vi "Average_IBP_curves_baseline_fromFile.vi"() -> ()   [LabVIEW 2015]
panel:
  in  "file path dn":path
  out "Resampled i(B) array":dbl[][](array[numeric])
  out "Mean I(B)":dbl[](array[numeric])
  out "XY Graph":cluster{dbl[], "Array out":dbl[]}[](graph)
  in  "Counter":i8
  in  "Min Field (T)":dbl
  in  "dB (T)":dbl=0.0025
  in  "Max Field (T)":dbl=0.15
  out "B array":dbl[](array[numeric])
  in  "file path (dialog if empty)":path
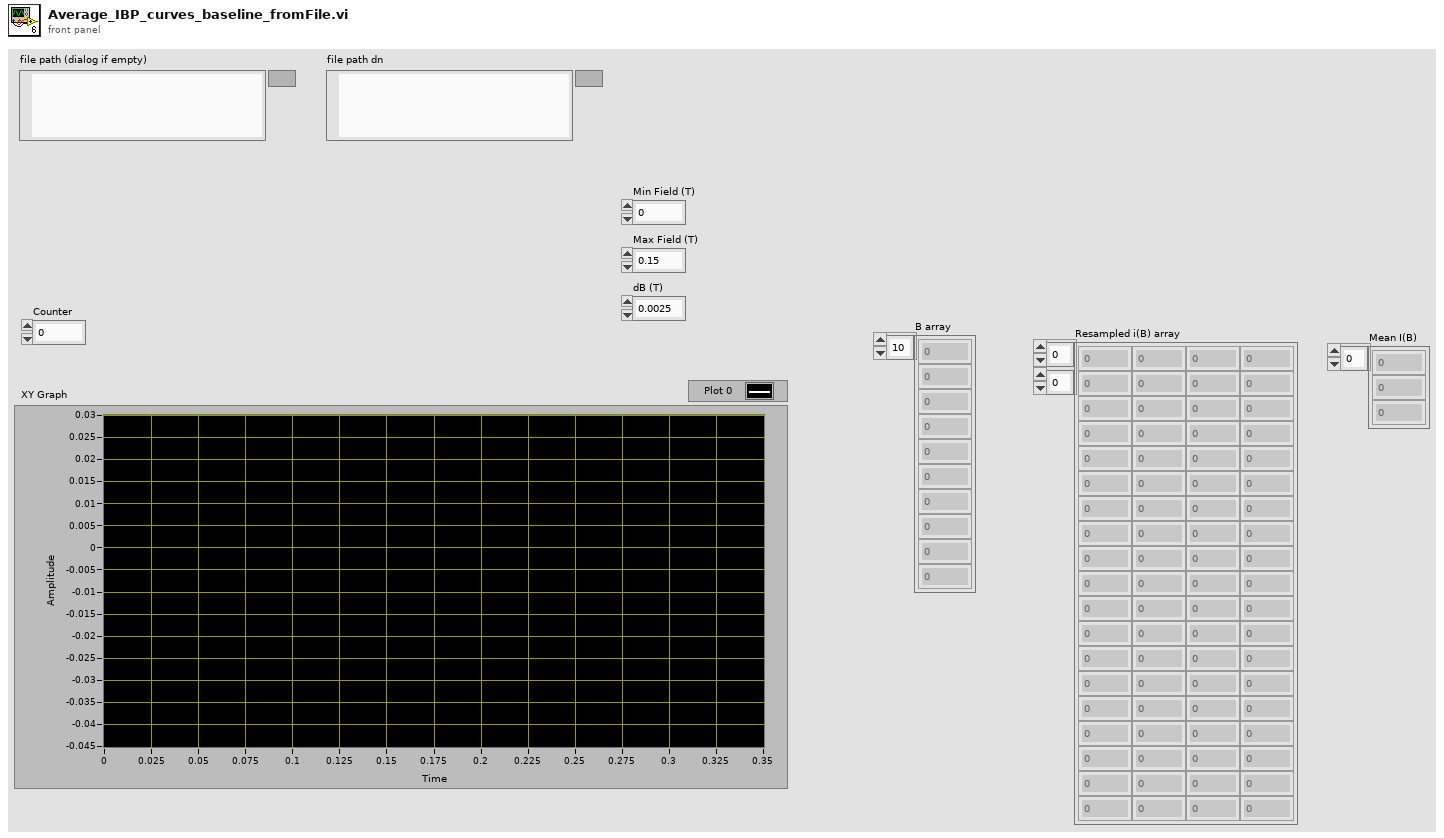
[diagram p1: front panel]
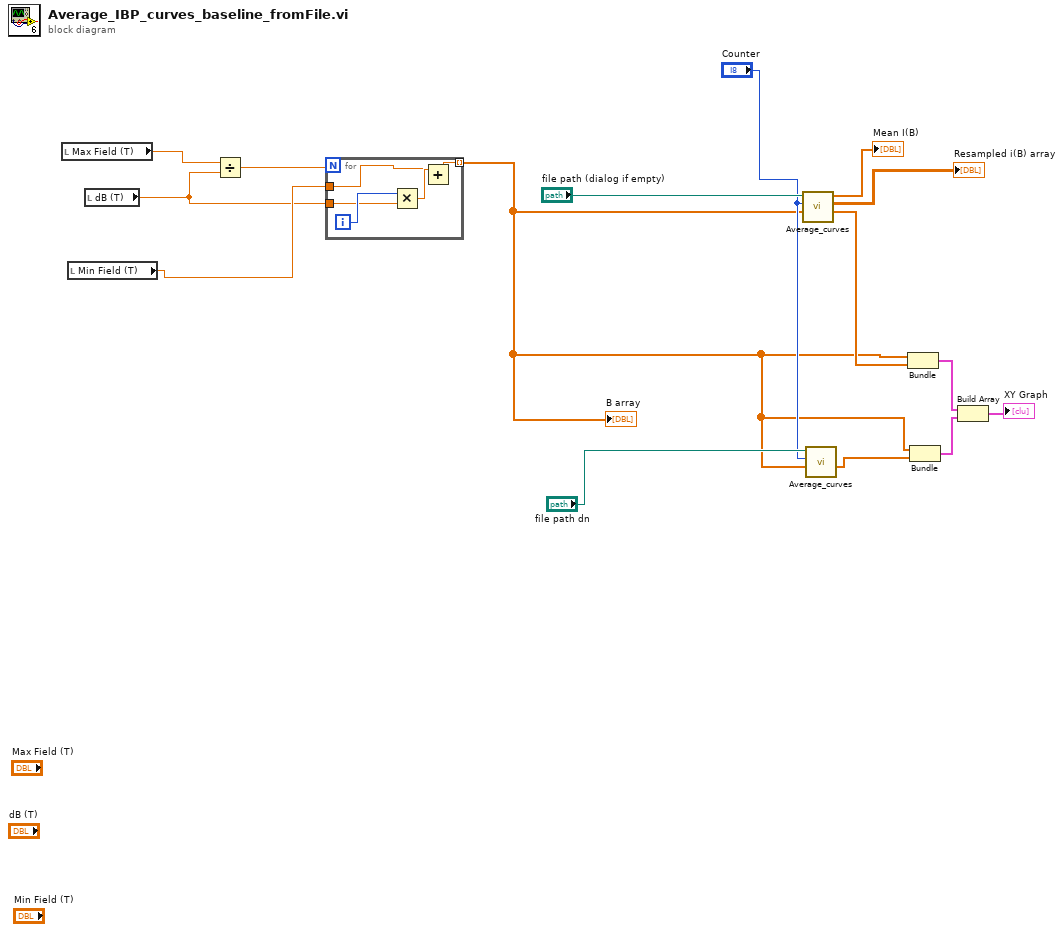
[diagram p0: block diagram]
diagram:
  n1 = local read "Max Field (T)"() -> (w11:dbl)
  n2 = local read "Min Field (T)"() -> (w13:dbl)
  n3 = local read "dB (T)"() -> (w12:dbl)
  n4 = Divide(x=w11, y=w12) -> (x/y=w14:dbl)
  n5 = for {
    N: w14 -> [_]
    tunnel: w12 -> [w19]
    tunnel: [w16] -> w5 mode=indexing
    tunnel: w13 -> [w17]
    i -> [w20]
    n6 = Multiply(x=w20, y=w19) -> (x*y=w18:dbl)
    n7 = Add(x=w18, y=w17) -> (x+y=w16:dbl)
  }
  "B array" <- w5
  n8 = call "Average_curves.vi"("Array in"=w5, "Counter"="Counter", "file path (dialog if empty)"="file path (dialog if empty)") -> ("Array out"=w10:dbl[], "Resampled i(B) array"=→"Resampled i(B) array":dbl[][], "Mean I(B)"=→"Mean I(B)":dbl[])  [unwired: 6 in]
  n9 = call "Average_curves.vi"("Array in"=w5, "Counter"="Counter", "file path (dialog if empty)"="file path dn") -> ("Array out"=w4:dbl[])  [unwired: 6 in, 2 out]
  n10 = Bundle(w5, "Array out"=w10) -> (w3:cluster{dbl[], "Array out":dbl[]})  [unwired: 1 in]
  n11 = Bundle(w5, "Array out"=w4) -> (w2:cluster{dbl[], "Array out":dbl[]})  [unwired: 1 in]
  n12 = Build Array(w3, w2) -> (→"XY Graph":cluster{dbl[], "Array out":dbl[]}[])
